vi "BackAndForthStepping.vi"() -> ()   [LabVIEW 2015]
uses:
  Common_RT_ILC/DataTypes/ILCTelemetry.ctl
  Common_RT_ILC/DataTypes/ILCScanRates.ctl
  Common_RT_ILC/DataTypes/ILCResponses.ctl
  Common_RT_Modbus/DataTypes/ExceptionCodes.ctl
  Common_RT_HPILC/DataTypes/HPResponses.ctl
  Common_RT_HPILC/DataTypes/HPTelemetry.ctl
  Common_RT_HealthAndStatus/RTHealthAndStatus/RTHealthAndStatus.lvclass
  MyHealthAndStatusReadFIFO/MyHealthAndStatusReadFIFO.lvclass
  MyHealthAndStatusWriteFIFO/MyHealthAndStatusWriteFIFO.lvclass
  ModbusFactory/ModbusFactory.lvclass
  SubnetFactory/SubnetFactory.lvclass
  Subnet/DataTypes/SubnetSettings.ctl
  Common_RT_HPILC/DataTypes/HPSettings.ctl
  Common_RT_ILC/DataTypes/ILCSettings.ctl
  Common_RT_Modbus/IModbusFactory/IModbusFactory.lvclass
  ModbusFactory/ModbusFactory.lvclass/ModbusFactory.ctl
  MyHealthAndStatusWriteFIFO/MyHealthAndStatusWriteFIFO.lvclass/MyHealthAndStatusWriteFIFO.ctl
  MyHealthAndStatusReadFIFO/MyHealthAndStatusReadFIFO.lvclass/MyHealthAndStatusReadFIFO.ctl
  Common_RT_HealthAndStatus/RTHealthAndStatus/RTHealthAndStatus.lvclass/RTHealthAndStatus.ctl
  Subnet/Subnet.lvclass/Subnet.ctl
  Common_RT_ILC/ILC/ILC.lvclass/ILC.ctl
  Common_RT_HPILC/HPILC/HPILC.lvclass/HPILC.ctl
  <vilib>/FPGAPlugInAG/cRIO-9038/niLvFpga_Open_cRIO-9038.vi
  <vilib>/rvi/interface/common/dynamic/niFpgaDynamicAddResources.vi
  <vilib>/FPGAPlugInAG/Dynamic/niLvFpga_Abort_Dynamic.vi
  <vilib>/FPGAPlugInAG/Dynamic/niLvFpga_Reset_Dynamic.vi
  <vilib>/FPGAPlugInAG/Dynamic/niLvFpga_Run_Dynamic.vi
  <vilib>/Utility/error.llb/Error Cluster From Error Code.vi
  <vilib>/rvi/errors/niLvFpgaAdjustHostInterfaceError.vi
  <vilib>/FPGAPlugInAG/Dynamic/niLvFpga_Close_Dynamic.vi
  <vilib>/rvi/interface/nirviOpenFPGA/nirviOpenFPGA.xnode
  FPGA Bitfiles/modbus1Port.lvbitx
  FPGA/main.vi
  <vilib>/rvi/interface/nirviMethod/nirviMethod.xnode
  <vilib>/rvi/interface/nirviCloseFPGA/nirviCloseFPGA.xnode
  Common_RT_ILC/RTILC.lvlib
  Common_RT_ILC/ILC/ILC.lvclass
  Common_RT_HPILC/RTHPILC.lvlib
  Common_RT_HPILC/HPILC/HPILC.lvclass
  Subnet/Subnet.lvclass
  <vilib>/rvi/errors/niLvFpgaMergeErrorWithErrorCode.vi
  <vilib>/FPGAPlugInAG/Dynamic/niLvFpga_ReadFifo_Dynamic.vi
  Common_RT_Modbus/RTModbus.lvlib
panel:
  out "Encoder":i32(graph)
  in  "Stop":bool
  out "HPTelemetry":T1
  out "HPResponses":T2 {"ForceAndStatus" items=["OK", "IllegalFunction", "IllegalDataAddress", "IllegalDataValue", "SlaveDeviceFailure", "Acknowledge", "SlaveDeviceBusy", "NegativeAcknowledge", "MemoryParityError", "GatewayPathUnavailable", "GatewayTargetDeviceFailedToRespond"]; "StepMotor" items=["OK", "IllegalFunction", "IllegalDataAddress", "IllegalDataValue", "SlaveDeviceFailure", "Acknowledge", "SlaveDeviceBusy", "NegativeAcknowledge", "MemoryParityError", "GatewayPathUnavailable", "GatewayTargetDeviceFailedToRespond"]}
  in  "Boolean":bool
  out "ILCResponses":T4 {"ADCOffsetSensitivity" items=["OK", "IllegalFunction", "IllegalDataAddress", "IllegalDataValue", "SlaveDeviceFailure", "Acknowledge", "SlaveDeviceBusy", "NegativeAcknowledge", "MemoryParityError", "GatewayPathUnavailable", "GatewayTargetDeviceFailedToRespond"]; "ADCScanRate" items=["OK", "IllegalFunction", "IllegalDataAddress", "IllegalDataValue", "SlaveDeviceFailure", "Acknowledge", "SlaveDeviceBusy", "NegativeAcknowledge", "MemoryParityError", "GatewayPathUnavailable", "GatewayTargetDeviceFailedToRespond"]; "Reset" items=["OK", "IllegalFunction", "IllegalDataAddress", "IllegalDataValue", "SlaveDeviceFailure", "Acknowledge", "SlaveDeviceBusy", "NegativeAcknowledge", "MemoryParityError", "GatewayPathUnavailable", "GatewayTargetDeviceFailedToRespond"]; "SetTemporaryAddress" items=["OK", "IllegalFunction", "IllegalDataAddress", "IllegalDataValue", "SlaveDeviceFailure", "Acknowledge", "SlaveDeviceBusy", "NegativeAcknowledge", "MemoryParityError", "GatewayPathUnavailable", "GatewayTargetDeviceFailedToRespond"]; "ILCMode" items=["OK", "IllegalFunction", "IllegalDataAddress", "IllegalDataValue", "SlaveDeviceFailure", "Acknowledge", "SlaveDeviceBusy", "NegativeAcknowledge", "MemoryParityError", "GatewayPathUnavailable", "GatewayTargetDeviceFailedToRespond"]; "ReportServerStatus" items=["OK", "IllegalFunction", "IllegalDataAddress", "IllegalDataValue", "SlaveDeviceFailure", "Acknowledge", "SlaveDeviceBusy", "NegativeAcknowledge", "MemoryParityError", "GatewayPathUnavailable", "GatewayTargetDeviceFailedToRespond"]; "ReportServerID" items=["OK", "IllegalFunction", "IllegalDataAddress", "IllegalDataValue", "SlaveDeviceFailure", "Acknowledge", "SlaveDeviceBusy", "NegativeAcknowledge", "MemoryParityError", "GatewayPathUnavailable", "GatewayTargetDeviceFailedToRespond"]}
  out "ILCTelemetry":T5 {"ADCScanRate" items=["50 Hz"=0, "60 Hz"=1, "100 Hz"=2, "120 Hz"=3, "200 Hz"=4, "240 Hz"=5, "300 Hz"=6, "400 Hz"=7, "480 Hz"=8, "600 Hz"=9, "1200 Hz"=10, "2400 Hz"=11, "4800 Hz"=12, "No Change"=255]}
  out "Port 1 Status Bits":u64 format="%016b"
  out "error out":errorcluster
  out "Port 1 Frames Received":i64
  out "Port 1 Bytes Received":i64
  out "Port 1 Frames Transmitted":i64
  out "Port 1 Bytes Transmitted":i64
  # "Port 1 = Modbus"
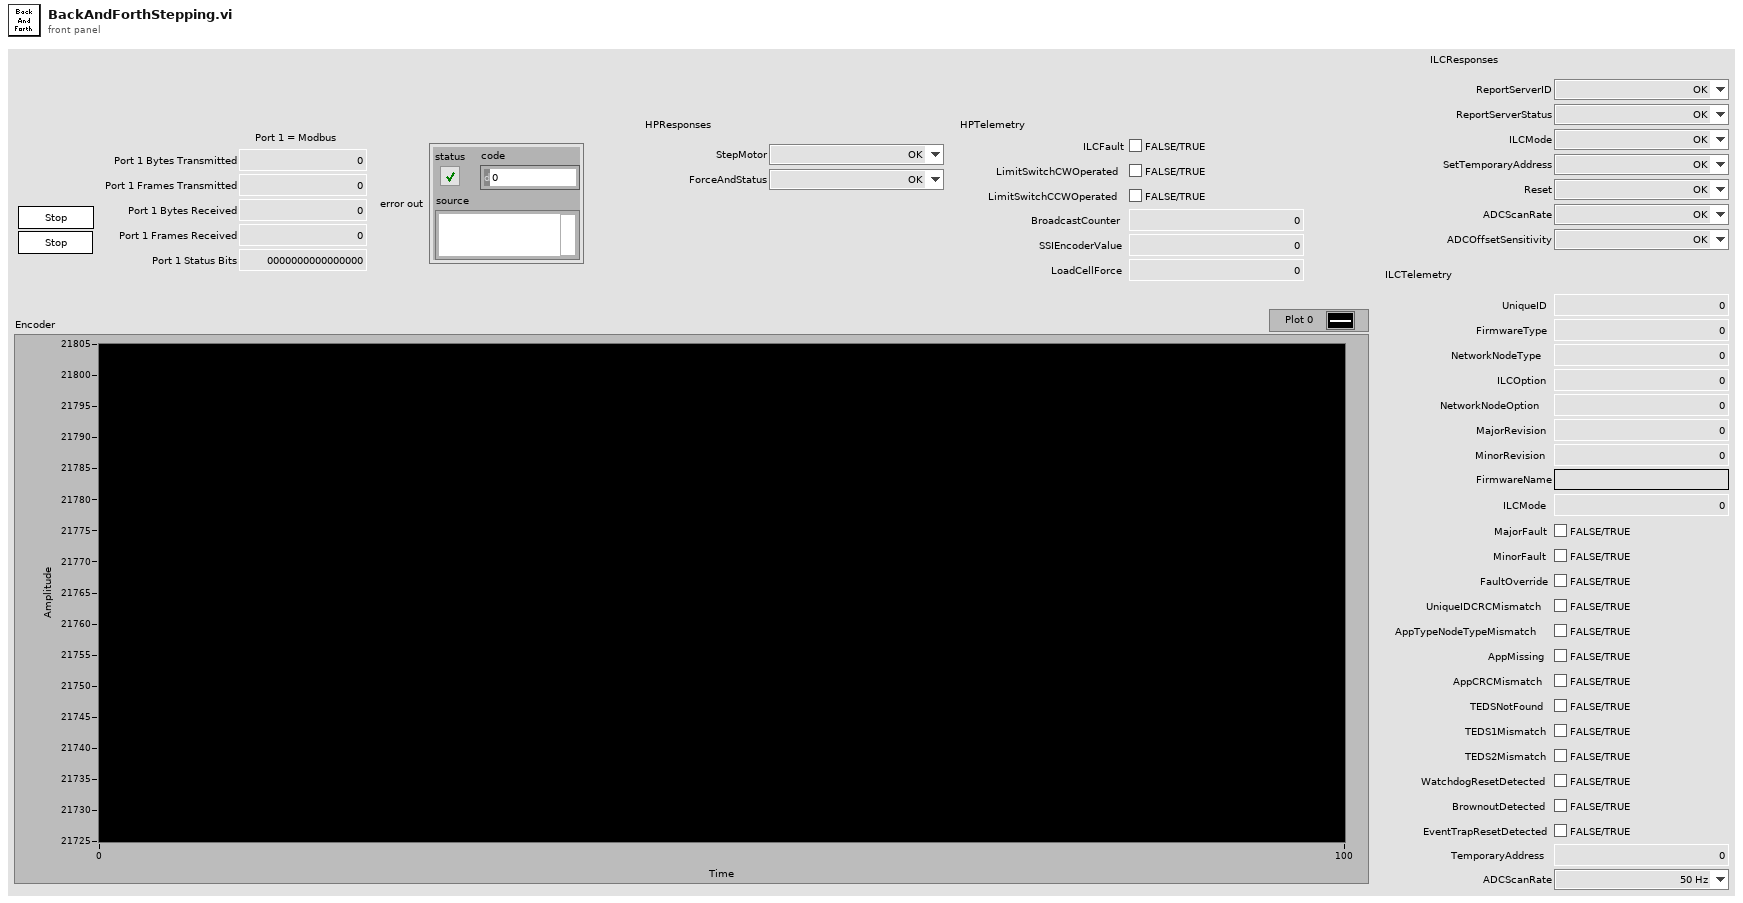
[diagram p1: front panel]
types:
  T1 = typedef "RTHPILC.lvlib/HPTelemetry.ctl" = cluster{"ILCFault":bool, "LimitSwitchCWOperated":bool, "LimitSwitchCCWOperated":bool, "BroadcastCounter":u8, "SSIEncoderValue":i32, "LoadCellForce":sgl}
  T2 = typedef "RTHPILC.lvlib/HPResponses.ctl" = cluster{"StepMotor":T3, "ForceAndStatus":T3}
  T3 = typedef "RTModbus.lvlib/ExceptionCodes.ctl" = u16
  T4 = typedef "RTILC.lvlib/ILCResponses.ctl" = cluster{"ReportServerID":T3, "ReportServerStatus":T3, "ILCMode":T3, "SetTemporaryAddress":T3, "Reset":T3, "ADCScanRate":T3, "ADCOffsetSensitivity":T3}
  T5 = typedef "RTILC.lvlib/ILCTelemetry.ctl" = cluster{"UniqueID":u64, "FirmwareType":u8, "NetworkNodeType":u8, "ILCOption":u8, "NetworkNodeOption":u8, "MajorRevision":u8, "MinorRevision":u8, "FirmwareName":string, "ILCMode":u16, "MajorFault":bool, "MinorFault":bool, "FaultOverride":bool, "UniqueIDCRCMismatch":bool, "AppTypeNodeTypeMismatch":bool, "AppMissing":bool, "AppCRCMismatch":bool, "TEDSNotFound":bool, "TEDS1Mismatch":bool, "TEDS2Mismatch":bool, "WatchdogResetDetected":bool, "BrownoutDetected":bool, "EventTrapResetDetected":bool, "TemporaryAddress":u8, "ADCScanRate":T6}
  T6 = typedef "RTILC.lvlib/ILCScanRates.ctl" = u8
  T7 = typedef "RTHPILC.lvlib/HPSettings.ctl" = cluster{"ILCSettings":T8, "ID":i16, "ReferencePosition":i32}
  T8 = typedef "RTILC.lvlib/ILCSettings.ctl" = cluster{"Subnet":u8, "Address":u8}
  T9 = typedef "SubnetSettings.ctl" = cluster{"HPs":T7[], "ModbusFactory":refnum<class "IModbusFactory.lvclass">, "Port":i32}
  T10 = typedef "SubnetData.ctl" = cluster{"SubnetConstants":T11, "SubnetCommand":T14, "SubnetTelemetry":T15}
  T11 = typedef "SubnetConstants.ctl" = cluster{"Modbus":refnum<class "IModbus.lvclass">, "HPs":refnum<class "HPILC.lvclass">[], "AddressToActuator":T12[]}
  T12 = typedef "ILCIndexData.ctl" = cluster{"ILCTypes":T13, "Index":i32}
  T13 = typedef "ILCTypes.ctl" = enum16{"Undefined", "SAA", "DAA", "HP"}
  T14 = typedef "SubnetCommand.ctl" = cluster{"BroadcastCounter":u8}
  T15 = typedef "SubnetTelemetry.ctl" = cluster{"BytesTransmitted":u32, "FramesTransmitted":u32, "BytesReceived":u32, "FramesReceived":u32, "TxInternalFIFOOverflow":bool, "InvalidInstruction":bool, "WaitForRxFrameTimeout":bool, "StartBitError":bool, "StopBitError":bool, "RxDataFIFOOverflow":bool}
  T16 = typedef "RTHPILC.lvlib/HPData.ctl" = cluster{"HPConstants":T17, "HPCommand":T18, "HPTelemetry":T1, "HPResponses":T2}
  T17 = typedef "RTHPILC.lvlib/HPConstants.ctl" = cluster{"ID":i16, "ReferencePosition":i32}
  T18 = typedef "RTHPILC.lvlib/HPCommand.ctl" = cluster{"Steps":i8}
  T19 = typedef "RTILC.lvlib/ILCData.ctl" = cluster{"Constants":T20, "Command":T21, "Telemetry":T5, "Responses":T4}
  T20 = typedef "RTILC.lvlib/ILCConstants.ctl" = cluster{"Subnet":u8, "Address":u8}
  T21 = typedef "RTILC.lvlib/ILCCommand.ctl" = cluster{"ILCMode":u16, "TemporaryAddress":u8, "ADCScanRate":T6, "ADCChannel":u8, "ADCOffset":sgl, "ADCSensitivity":sgl}
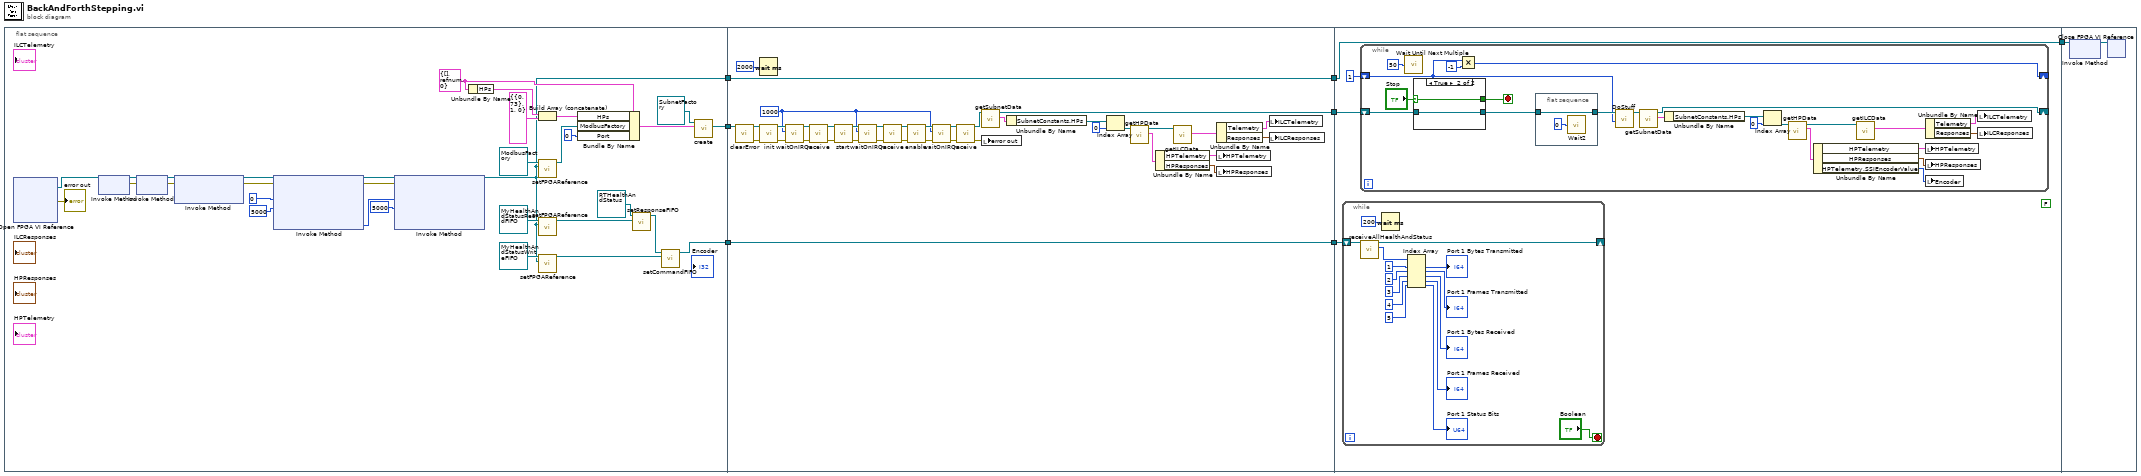
[diagram p0: block diagram]
diagram:
  n1 = flat-sequence {
    tunnel: [w10] -> w7
    tunnel: [w36] -> w4
    tunnel: [w20] -> w2
    tunnel: w7 -> [w76]
    tunnel: [w76] -> w6
    tunnel: w4 -> [w74]
    tunnel: [w74] -> w3
    tunnel: w2 -> [w42]
    tunnel: [w44] -> w1
    tunnel: w6 -> [w79]
    tunnel: [w79] -> w5
    tunnel: w3 -> [w80]
    tunnel: w1 -> [w78]
    tunnel: w5 -> [w125]
    frame #0 {
      w25 = T9 {"HPs"=[], "ModbusFactory"=refnum, "Port"=0} ("SubnetSettings")
      n2 = xnode "Open FPGA VI Reference"() -> ("FPGA VI Reference Out"=w30:refnum<k20>, "error out"=→"error out":errorcluster)  [unwired: 2 in]
      n3 = xnode "Invoke Method"("FPGA VI Reference In"=w30) -> ("FPGA VI Reference Out"=w39:refnum<k20>, "error out"=w31:errorcluster)  [unwired: 1 in]
      n4 = xnode "Invoke Method"("FPGA VI Reference In"=w39, "error in"=w31) -> ("FPGA VI Reference Out"=w12:refnum<k20>, "error out"=w9:errorcluster)
      n5 = xnode "Invoke Method"("FPGA VI Reference In"=w12, "error in"=w9) -> ("FPGA VI Reference Out"=w11:refnum<k20>, "error out"=w8:errorcluster)  [unwired: 1 in]
      n6 = xnode "Invoke Method"("FPGA VI Reference In"=w11, "error in"=w8, "Number of Elements"=u32 0, "Timeout (ms)"=5000) -> ("FPGA VI Reference Out"=w15:refnum<k20>, "error out"=w13:errorcluster, "Elements Remaining"=w16:u32)  [unwired: 1 out]
      n7 = xnode "Invoke Method"("FPGA VI Reference In"=w15, "error in"=w13, "Number of Elements"=w16, "Timeout (ms)"=5000) -> ("FPGA VI Reference Out"=w10:refnum<k20>)  [unwired: 3 out]
      n8 = Unbundle By Name(w25) -> ("HPs"=w27:T7[])
      n9 = Build Array (concatenate)(w27, T7 {"ILCSettings"={"Subnet"=0, "Address"=73}, "ID"=1, "ReferencePosition"=0} ("HPSettings")) -> (w19:T7[])
      n10 = call "setFPGAReference.vi"("FPGAReference"=w10, "ModbusFactory in"=refnum<class "ModbusFactory.lvclass"> refnum ("ModbusFactory.lvclass")) -> ("ModbusFactory out"=w23:refnum<class "ModbusFactory.lvclass">)  [unwired: 9 in]
      n11 = call "setFPGAReference.vi"("FPGAReference"=w10, "MyHealthAndStatusReadFIFO in"=refnum<class "MyHealthAndStatusReadFIFO.lvclass"> refnum ("MyHealthAndStatusReadFIFO.lvclass")) -> ("MyHealthAndStatusReadFIFO out"=w34:refnum<class "MyHealthAndStatusReadFIFO.lvclass">)  [unwired: 9 in]
      n12 = call "setFPGAReference.vi"("FPGAReference"=w10, "MyHealthAndStatusWriteFIFO in"=refnum<class "MyHealthAndStatusWriteFIFO.lvclass"> refnum ("MyHealthAndStatusWriteFIFO.lvclass")) -> ("MyHealthAndStatusWriteFIFO out"=w32:refnum<class "MyHealthAndStatusWriteFIFO.lvclass">)  [unwired: 9 in]
      n13 = Bundle By Name(cluster=w25, "HPs"=w19, "ModbusFactory"=w23, "Port"=0) -> (w22:T9)
      n14 = call "setResponseFIFO.vi"("ReadU32FIFO"=w34, "RTHealthAndStatus in"=refnum<class "RTHealthAndStatus.lvclass"> refnum ("RTHealthAndStatus.lvlib:RTHealthAndStatus.lvclass")) -> ("RTHealthAndStatus out"=w37:refnum<class "RTHealthAndStatus.lvclass">)  [unwired: 9 in]
      n15 = call "setCommandFIFO.vi"("WriteU64FIFO"=w32, "RTHealthAndStatus in"=w37) -> ("RTHealthAndStatus out"=w36:refnum<class "RTHealthAndStatus.lvclass">)  [unwired: 9 in]
      n16 = call "create.vi"("SubnetSettings"=w22, "SubnetFactory in"=refnum<class "SubnetFactory.lvclass"> refnum ("SubnetFactory.lvclass")) -> ("Subnet"=w20:refnum<class "Subnet.lvclass">)  [unwired: 7 in, 2 out]
    }
    frame #1 {
      w57 = 1000 ("Timeout (ms)")
      n17 = call "clearError.vi"("Subnet in"=w42) -> ("error out"=w40:errorcluster, "Subnet out"=w41:refnum<class "Subnet.lvclass">)  [unwired: 9 in]
      n18 = Wait (ms)(milliseconds to wait=u32 2000) -> ()  [unwired: 1 out]
      n19 = call "init.vi"("error in (no error)"=w40, "Subnet in"=w41) -> ("error out"=w70:errorcluster, "Subnet out"=w73:refnum<class "Subnet.lvclass">)  [unwired: 8 in]
      n20 = call "waitOnIRQs.vi"("error in (no error)"=w70, "Timeout (ms)"=w57, "Subnet in"=w73) -> ("error out"=w71:errorcluster, "Subnet out"=w72:refnum<class "Subnet.lvclass">)  [unwired: 7 in]
      n21 = call "receive.vi"("error in (no error)"=w71, "Subnet in"=w72) -> ("error out"=w67:errorcluster, "Subnet out"=w69:refnum<class "Subnet.lvclass">)  [unwired: 8 in]
      n22 = call "start.vi"("error in (no error)"=w67, "Subnet in"=w69) -> ("error out"=w66:errorcluster, "Subnet out"=w68:refnum<class "Subnet.lvclass">)  [unwired: 8 in]
      n23 = call "waitOnIRQs.vi"("error in (no error)"=w66, "Timeout (ms)"=w57, "Subnet in"=w68) -> ("error out"=w64:errorcluster, "Subnet out"=w65:refnum<class "Subnet.lvclass">)  [unwired: 7 in]
      n24 = call "receive.vi"("error in (no error)"=w64, "Subnet in"=w65) -> ("error out"=w62:errorcluster, "Subnet out"=w63:refnum<class "Subnet.lvclass">)  [unwired: 8 in]
      n25 = call "enable.vi"("error in (no error)"=w62, "Subnet in"=w63) -> ("error out"=w58:errorcluster, "Subnet out"=w61:refnum<class "Subnet.lvclass">)  [unwired: 8 in]
      n26 = call "waitOnIRQs.vi"("error in (no error)"=w58, "Timeout (ms)"=w57, "Subnet in"=w61) -> ("error out"=w60:errorcluster, "Subnet out"=w59:refnum<class "Subnet.lvclass">)  [unwired: 7 in]
      n27 = call "receive.vi"("error in (no error)"=w60, "Subnet in"=w59) -> ("error out"=w43:errorcluster, "Subnet out"=w56:refnum<class "Subnet.lvclass">)  [unwired: 8 in]
      n28 = call "getSubnetData.vi"("Subnet in"=w56) -> ("SubnetData"=w55:T10, "Subnet out"=w44:refnum<class "Subnet.lvclass">)  [unwired: 9 in]
      n29 = local write "error out"(w43) -> ()
      n30 = Unbundle By Name(w55) -> ("SubnetConstants.HPs"=w54:refnum<class "HPILC.lvclass">[])
      n31 = Index Array(array=w54, index=0) -> (element=w52:refnum<class "HPILC.lvclass">)
      n32 = call "getHPData.vi"("HardPointActuator in"=w52) -> ("HPData"=w48:T16, "HardPointActuator out"=w51:refnum<class "HPILC.lvclass">)  [unwired: 9 in]
      n33 = Unbundle By Name(w48) -> ("HPTelemetry"=w50:T1, "HPResponses"=w49:T2)
      n34 = call "getILCData.vi"("ILC in"=w51) -> ("ILCData"=w45:T19)  [unwired: 9 in, 1 out]
      n35 = Unbundle By Name(w45) -> ("Telemetry"=w47:T5, "Responses"=w46:T4)
      n36 = local write "HPTelemetry"(w50) -> ()
      n37 = local write "HPResponses"(w49) -> ()
      n38 = local write "ILCTelemetry"(w47) -> ()
      n39 = local write "ILCResponses"(w46) -> ()
    }
    frame #2 {
      (unwired) FALSE
      n40 = while {
        shift-right: [w122] -> _
        shift-left: w80 -> [w123]
        stop <- "Boolean" stop-if-true
        n41 = call "receiveAllHealthAndStatus.vi"("RTHealthAndStatus in"=w123) -> ("Data"=w117:u32[], "RTHealthAndStatus out"=w122:refnum<class "RTHealthAndStatus.lvclass">)  [unwired: 8 in, 1 out]
        n42 = Wait (ms)(milliseconds to wait=u32 200) -> ()  [unwired: 1 out]
        n43 = Index Array(array=w117, index #1=1 ("index"), index #2=2 ("index"), index #3=3 ("index"), index #4=4 ("index"), index #5=5 ("index")) -> (element #1=→"Port 1 Bytes Transmitted":u32, element #2=→"Port 1 Frames Transmitted":u32, element #3=→"Port 1 Bytes Received":u32, element #4=→"Port 1 Frames Received":u32, element #5=→"Port 1 Status Bits":u32)
      }
      n44 = while {
        shift-right: [w83] -> _
        shift-left: w78 -> [w101]
        shift-right: [w82] -> _
        shift-left: 1 -> [w85]
        stop <- w102 stop-if-true
        n45 = call "Wait Until Next Multiple"("Count(mSec)"=u32 50) -> ()  [unwired: 1 out]
        n46 = case shown="True" "Stop" {
          selector: "Stop" -> [w106 w108]
          tunnel: [w106 w108] -> w102
          tunnel: w101 -> [w107 w109]
          tunnel: [w107 w109] -> w100
          frame False {
          }
          frame True {
          }
        }
        n47 = Multiply(x=w85, y=-1) -> (x*y=w82:i32)
        n48 = flat-sequence {
          tunnel: w100 -> [w104]
          tunnel: [w104] -> w86
          frame #0 {
            n49 = call "Wait2"("Count(mSec)"=u32 0) -> ()  [unwired: 1 out]
          }
        }
        n50 = call "DoStuff.vi"("Steps"=w85, "Subnet in"=w86) -> ("Subnet out"=w94:refnum<class "Subnet.lvclass">)  [unwired: 7 in, 2 out]
        n51 = call "getSubnetData.vi"("Subnet in"=w94) -> ("SubnetData"=w96:T10, "Subnet out"=w83:refnum<class "Subnet.lvclass">)  [unwired: 9 in]
        n52 = Unbundle By Name(w96) -> ("SubnetConstants.HPs"=w97:refnum<class "HPILC.lvclass">[])
        n53 = Index Array(array=w97, index=0) -> (element=w99:refnum<class "HPILC.lvclass">)
        n54 = call "getHPData.vi"("HardPointActuator in"=w99) -> ("HPData"=w93:T16, "HardPointActuator out"=w95:refnum<class "HPILC.lvclass">)  [unwired: 9 in]
        n55 = Unbundle By Name(w93) -> ("HPTelemetry"=w89:T1, "HPResponses"=w88:T2, "HPTelemetry.SSIEncoderValue"=w87:i32)
        n56 = call "getILCData.vi"("ILC in"=w95) -> ("ILCData"=w92:T19)  [unwired: 9 in, 1 out]
        n57 = Unbundle By Name(w92) -> ("Telemetry"=w91:T5, "Responses"=w90:T4)
        n58 = local write "HPTelemetry"(w89) -> ()
        n59 = local write "HPResponses"(w88) -> ()
        n60 = local write "Encoder"(w87) -> ()
        n61 = local write "ILCTelemetry"(w91) -> ()
        n62 = local write "ILCResponses"(w90) -> ()
      }
    }
    frame #3 {
      n63 = xnode "Invoke Method"("FPGA VI Reference In"=w125) -> ("FPGA VI Reference Out"=w126:refnum<k20>)  [unwired: 1 in, 1 out]
      n64 = xnode "Close FPGA VI Reference"("FPGA VI Reference In"=w126) -> ()  [unwired: 1 in, 1 out]
    }
  }
